vi "4461 - Cal Info.vi"(8 "error in (no error)":errorcluster, 9 "Perform Auto Calibration":bool, 10 "Refnum In 2":refnum<k21>[](array[refnum]), 11 "Refnum In":refnum<k21>[](array[refnum])) -> (0 "error out":errorcluster, 2 "Cal Info":T1(array[cluster]))   [LabVIEW 2016]
uses:
  <vilib>/addons/WireFlow/_WF_ProgressBar.llb/WindowBehavior.ctl
  <userlib>/_OpenG.lib/array/array.llb/Remove Duplicates from 1D Array (String)__ogtk.vi
  <vilib>/addons/WireFlow/_WF_ProgressBar.llb/ProgressBar_WireFlow.lvclass
  <resource>/objmgr/daqmx.rc
panel:
  out "Numeric":i32
  out "dev temp >5°C from cal temp":bool
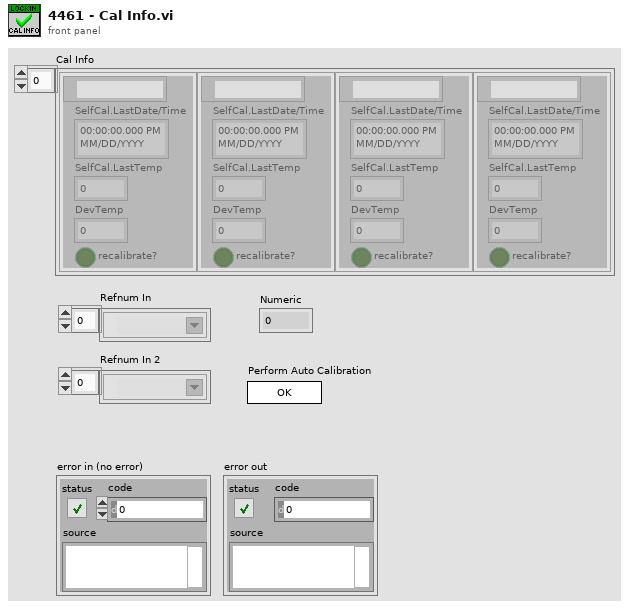
[diagram p1: front panel]
types:
  T1 = cluster{tag, "SelfCal.LastDate/Time":timestamp, "SelfCal.LastTemp":dbl, "DevTemp":dbl, "recalibrate?":bool}[]
  T2 = typedef "ProgressBar_WireFlow.lvclass/WindowBehavior.ctl" = enum16{"No change", "Modal", "Floating"}
  T3 = cluster{"String":string, "SelfCal.LastDate/Time":timestamp, "SelfCal.LastTemp":dbl, "DevTemp":dbl, bool}
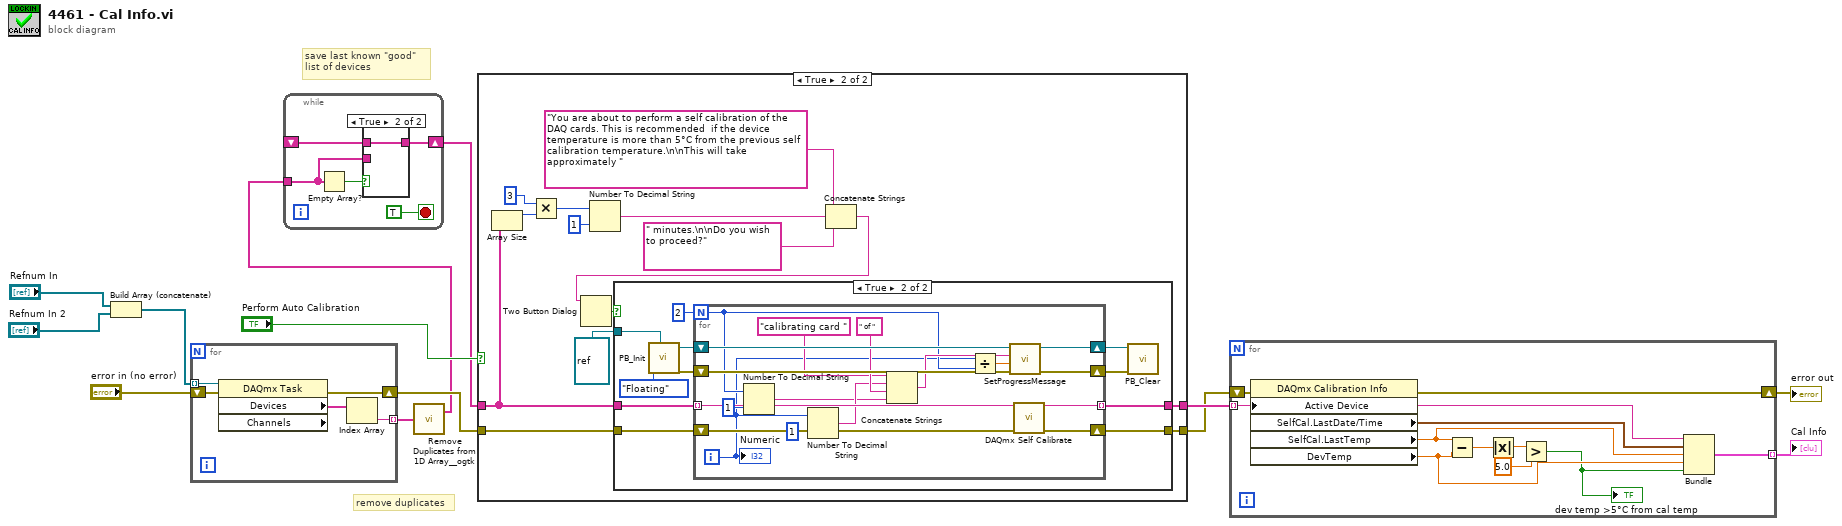
[diagram p0: block diagram]
diagram:
  # "save last known \"good\"\nlist of devices"
  # "remove duplicates"
  n1 = Build Array (concatenate)("Refnum In", "Refnum In 2") -> (w10:refnum<k21>[])
  n2 = for {
    tunnel: [w16] -> w9 mode=indexing
    shift-right: [w17] -> w6
    shift-left: "error in (no error)" -> [w18]
    tunnel: w10 -> [w14] mode=indexing
    n3 = property class="DAQmx Task" props=["Devices", "Channels"](reference=w14, error in=w18) -> (error out=w17:errorcluster, "Devices"=w15:tag[])  [unwired: 2 out]
    n4 = Index Array(array=w15) -> (element=w16:tag)  [unwired: 1 in]
  }
  n5 = call-poly <userlib>:"Remove Duplicates from 1D Array__ogtk.vi"("Input Array"=w9) -> ("Output Array"=w2:string[])  [unwired: 1 out]
  n6 = while {
    shift-right: [w21] -> w1
    shift-left: _ -> [w19]
    tunnel: w2 -> [w20]
    stop <- TRUE stop-if-true
    n7 = Empty Array?(array=w20) -> (empty?=w22:bool)
    n8 = case shown="True" w22 {
      tunnel: [w24 w25] -> w21
      tunnel: w20 -> [w24 _]
      tunnel: w19 -> [_ w25]
      frame False {
      }
      frame True {
      }
    }
  }
  n9 = case shown="True" "Perform Auto Calibration" {
    tunnel: w6 -> [w27 w41]
    tunnel: [w27 w40] -> w4
    tunnel: w1 -> [w26 w38]
    tunnel: [w26 w39] -> w5
    frame False {
    }
    frame True {
      n10 = Array Size(array=w38) -> (size(s)=w37:i32)
      n11 = Multiply(x=3, y=w37) -> (x*y=w29:i32)
      n12 = Number To Decimal String(number=w29, width (-)=i16 1) -> (decimal integer string=w30:string)
      n13 = Concatenate Strings("You are about to perform a self calibration of the DAQ cards. This is recommended  if the device temperature is more than 5°C from the previous self calibration temperature.\n\nThis will take approximately " ("message"), w30, " minutes.\n\nDo you wish to proceed?") -> (w31:string)
      n14 = Two Button Dialog(message=w31) -> (T button?=w32:bool)  [unwired: 2 in]
      n15 = case shown="True" w32 {
        tunnel: w41 -> [w43 w54]
        tunnel: [w43 w53] -> w40
        tunnel: [w42 w52] -> w39
        tunnel: w38 -> [w42 w51]
        tunnel: refnum<vi> refnum ("Progress VI") -> [_ w46]
        frame False {
        }
        frame True {
          n16 = call <vilib>:"PB_Init.vi"("Progress VI"=w46, "Window behavior (No change)"=WindowBehavior."Floating") -> ("error out"=w47:errorcluster, "WF-ProgressBar out"=w48:refnum<class "ProgressBar_WireFlow.lvclass">)  [unwired: 8 in]
          n17 = for {
            N: 2 -> [w60]
            shift-right: [w70] -> w53
            shift-left: w54 -> [w71]
            tunnel: w51 -> [w69] mode=indexing
            tunnel: [w69] -> w52 mode=indexing
            shift-right: [w66] -> w50
            shift-left: w48 -> [w67]
            shift-right: [w65] -> w49
            shift-left: w47 -> [w68]
            i -> [w55]
            n18 = Number To Decimal String(number=w60, width (-)=i16 1) -> (decimal integer string=w56:string)
            n19 = Number To Decimal String(number=w55, width (-)=i16 1) -> (decimal integer string=w58:string)
            n20 = Concatenate Strings("calibrating card ", w58, " of ", w56) -> (w61:string)
            n21 = Divide(x=w55, y=w60) -> (x/y=w62:dbl)
            n22 = call-dynamic "SetProgressMessage.vi"("error in (no error)"=w68, "Progress value (NaN no update)"=w62, "Message"=w61, "WF-ProgressBar in"=w67) -> ("error out"=w65:errorcluster, "WF-ProgressBar out"=w66:refnum<class "ProgressBar_WireFlow.lvclass">)  [unwired: 5 in, 1 out]
            n23 = call <vilib>:"DAQmx Self Calibrate.vi"("device in"=w69, "error in"=w71) -> ("error out"=w70:errorcluster)  [unwired: 13 in]
            "Numeric" <- w55
          }
          n24 = call-dynamic "PB_Clear.vi"("error in (no error)"=w49, "WF-ProgressBar in"=w50) -> ()  [unwired: 8 in, 2 out]
        }
      }
    }
  }
  n25 = for {
    tunnel: [w81] -> w7 mode=indexing
    shift-right: [w82] -> w8
    shift-left: w4 -> [w80]
    tunnel: w5 -> [w72] mode=indexing
    n26 = property class="DAQmx Calibration Info"(error in=w80, "Active Device"=w72) -> (error out=w82:errorcluster, "SelfCal.LastDate/Time"=w76:timestamp, "SelfCal.LastTemp"=w75:dbl, "DevTemp"=w74:dbl)  [unwired: 1 in, 1 out]
    n27 = Subtract(x=w75, y=w74) -> (x-y=w79:dbl)
    n28 = Absolute Value(x=w79) -> (abs(x)=w78:dbl)
    n29 = Greater?(x=w78, y=5.0) -> (0:w73:bool)
    "dev temp >5°C from cal temp" <- w73
    n30 = Bundle("String"=w72, "SelfCal.LastDate/Time"=w76, "SelfCal.LastTemp"=w75, "DevTemp"=w74, w73) -> (w81:T3)  [unwired: 1 in]
  }
  "error out" <- w8
  "Cal Info" <- w7
